vi "ExFileReadNConvertToDatatype.vi"() -> ()   [LabVIEW 2010]
panel:
  in  "Output file name":path=path "C:/Program Files/SIToolKit/LabVIEW/Data Files/test"
  in  "data type":u32=7 min=1 max=8 step=1
  in  "Full File Name":path=path "C:/Program Files/SIToolKit/LabVIEW/Data Files/Color.SPE"
  in  "?":bool
  in  "FileType":u32=67371008
  out "error out":errorcluster
  in  "error in (no error)":errorcluster
  # "ExReadFileNconvertToDatatype.vi\nThis example will read in a file of the\nselected data type and display as datatype frame.\nWhen finished viewing data, make sure to\nuse the STOP button to close the display."
  # "File Types:\nSPE = 67371008\nTIF   = 67174400\nPMI  = 67436544"
  # "Browse match pattern is set to *.spe.  Modify this if different file type is needed."
  # "NOTICE\n\nTHIS VI REQUIRES THAT THE TOOLKIT\nBE UNLOADED BY RUNNING THE\n VI EXCLOSEGLOBALCAM.VI\n BEFORE LEAVING LABVIEW."
  # "This will properly close\nthe image and\ndeallocate memory."
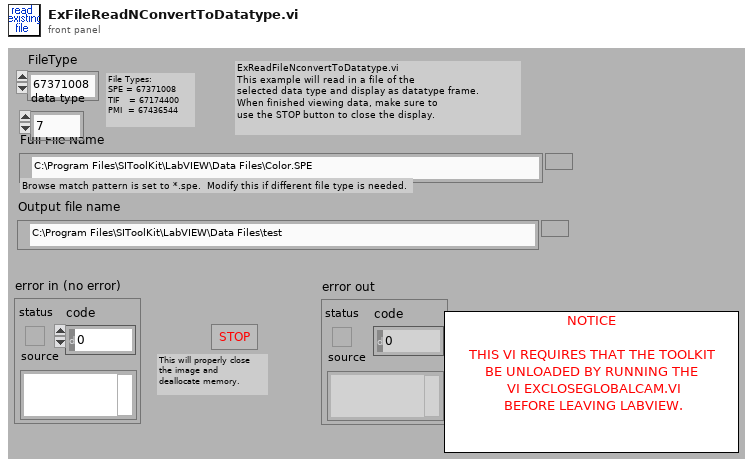
[diagram p1: front panel]
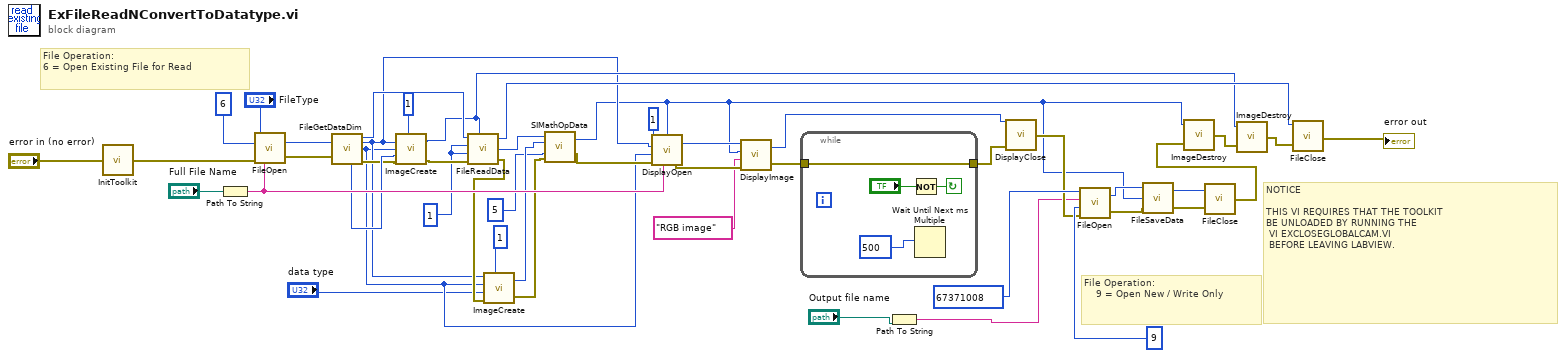
[diagram p0: block diagram]
diagram:
  w35 = 1
  # "NOTICE\n\nTHIS VI REQUIRES THAT THE TOOLKIT\nBE UNLOADED BY RUNNING THE\n VI EXCLOSEGLOBALCAM.VI\n BEFORE LEAVING LABVIEW."
  # "File Operation:\n    9 = Open New / Write Only"
  # "File Operation:\n6 = Open Existing File for Read"
  n1 = call <userlib>:"InitToolkit.vi"("error in"="error in (no error)") -> ("error out"=w45:errorcluster)
  n2 = Path To String(path="Full File Name") -> (string=w38:string)
  n3 = call <userlib>:"FileOpen.vi"("error in"=w45, "File Operations"=u32 6 ("File Operation"), "FileName"=w38, "File Type"="FileType") -> ("error out"=w43:errorcluster, "File Handle"=w42:u32)
  n4 = call <userlib>:"FileGetDataDim.vi"("File Handle"=w42, "error in"=w43) -> ("Data Type"=w25:u32, "File Handle"=w37:u32, "X dim"=w7:u32, "Y dim"=w6:u32, "error out"=w22:errorcluster)  [unwired: 1 out]
  n5 = call <userlib>:"ImageCreate.vi"("X dimension"=w7, "Y dimension"=w6, "Data Type"=w25, "error in"=w22, "Number Of Frames"=1) -> ("Image Handle"=w27:u32, "error out"=w36:errorcluster)
  n6 = call <userlib>:"FileReadData.vi"("File Handle"=w37, "Start Frame"=w35, "End Frame"=w35, "error in"=w36, "Image Handle"=w27) -> ("File Handle"=w34:u32, "Image Handle"=w19:u32, "error out"=w23:errorcluster)
  n7 = call <userlib>:"ImageCreate.vi"("X dimension"=w7, "Y dimension"=w6, "Data Type"="data type", "error in"=w23, "Number Of Frames"=1) -> ("Image Handle"=w20:u32, "error out"=w21:errorcluster)
  n8 = call <userlib>:"SIMathOpData.vi"("error in (no error)"=w21, "Operation"=5, "Result Handle"=w20, "Data Handle"=w19) -> ("error out"=w17:errorcluster, "Result Handle"=w5:u32)
  n9 = call <userlib>:"DisplayOpen.vi"("Display Title"=w38, "Image Handle"=w5, "error in"=w17, "Display Height"=w6, "Display Width"=w7, "Display Type"=1) -> ("error out"=w33:errorcluster, "Display Handle"=w32:u32)
  n10 = call <userlib>:"DisplayImage.vi"("error in"=w33, "Title"="RGB image", "Image Handle"=w5, "Display Handle"=w32) -> ("error out"=w26:errorcluster, "Display Handle"=w31:u32)
  n11 = while {
    tunnel: w26 -> [w48]
    tunnel: [w48] -> w10
    stop <- w50 continue-if-true
    n12 = Not(x="?") -> (.not. x?=w50:bool)
    n13 = Wait Until Next ms Multiple(millisecond multiple=500) -> ()  [unwired: 1 out]
  }
  n14 = Path To String(path="Output file name") -> (string=w2:string)
  n15 = call <userlib>:"DisplayClose.vi"("error in"=w10, "Display Handle"=w31) -> ("error out"=w9:errorcluster)
  n16 = call <userlib>:"FileOpen.vi"("error in"=w9, "File Operations"=9, "FileName"=w2, "File Type"=67371008) -> ("error out"=w16:errorcluster, "File Handle"=w14:u32)
  n17 = call <userlib>:"FileSaveData.vi"("error in"=w16, "Image Handle"=w5, "File Handle"=w14) -> ("error out"=w15:errorcluster, "File Handle"=w13:u32)
  n18 = call <userlib>:"FileClose.vi"("error in"=w15, "File Handle"=w13) -> ("error out"=w8:errorcluster)
  n19 = call <userlib>:"ImageDestroy.vi"("error in"=w8, "Data handle"=w5) -> ("error out"=w30:errorcluster)
  n20 = call <userlib>:"ImageDestroy.vi"("error in"=w30, "Data handle"=w27) -> ("error out"=w29:errorcluster)
  n21 = call <userlib>:"FileClose.vi"("error in"=w29, "File Handle"=w34) -> ("error out"=→"error out":errorcluster)
